vi "DAC set voltage.vi"(8 "Calibration array":dbl[][](array[numeric]), 10 "DAC output (V)":dbl, 11 "VISA Refnum in":refnum<visa-resource-name>) -> (3 "VISA Refnum out":refnum<visa-resource-name>, 6 "Output code":u16)   [LabVIEW 2015]
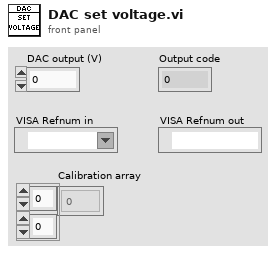
[diagram p1: front panel]
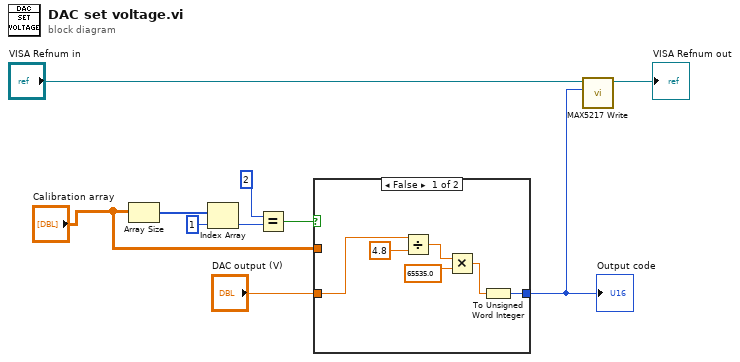
[diagram p0: block diagram]
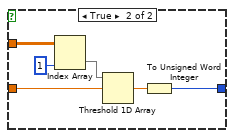
[diagram p2: hidden frame]
diagram:
  n1 = Array Size(array="Calibration array") -> (size(s)=w5:i32[])
  n2 = Index Array(array=w5, index=1) -> (element=w7:i32)
  n3 = Equal?(x=2, y=w7) -> (x = y?=w4:bool)
  n4 = case shown="False" w4 {
    tunnel: "DAC output (V)" -> [w12 w22]
    tunnel: [w11 w20] -> w2
    tunnel: "Calibration array" -> [_ w19]
    frame False {
      n5 = Divide(x=w12, y=4.8) -> (x/y=w13:dbl)
      n6 = Multiply(x=w13, y=65535.0) -> (x*y=w16:dbl)
      n7 = To Unsigned Word Integer(number=w16) -> (unsigned 16bit integer=w11:u16)
    }
    frame True {
      n8 = Index Array(array=w19, index (col)=1 ("disabled index (col)")) -> (element=w18:dbl[])  [unwired: 1 in]
      n9 = Threshold 1D Array(2:w22, 3:w18) -> (0:w21:dbl)  [unwired: 1 in]
      n10 = To Unsigned Word Integer(number=w21) -> (unsigned 16bit integer=w20:u16)
    }
  }
  "Output code" <- w2
  n11 = call "MAX5217 Write.vi"("DAC code"=w2, "VISA Refnum in"="VISA Refnum in") -> ("VISA Refnum out"=→"VISA Refnum out":refnum<visa-resource-name>)  [unwired: 6 in, 1 out]
